vi "Create.vi"(8 "error in (no error)":errorcluster caption="错误输入（无错误）") -> (0 "error out":errorcluster caption="错误输出", 3 "ImageListClass 输出":refnum<class "ImageListClass.lvclass"> caption="DNL_LabVIEW Object out")   [LabVIEW 2013, in "ImageListClass.lvclass"]
uses:
  ImageListClass.lvclass
  System.Windows.Forms
  ImageListClass.lvclass/ImageListClass.ctl
panel:
  in  "ImageListClass 输入":refnum<class "ImageListClass.lvclass"> caption="DNL_LabVIEW Object in"
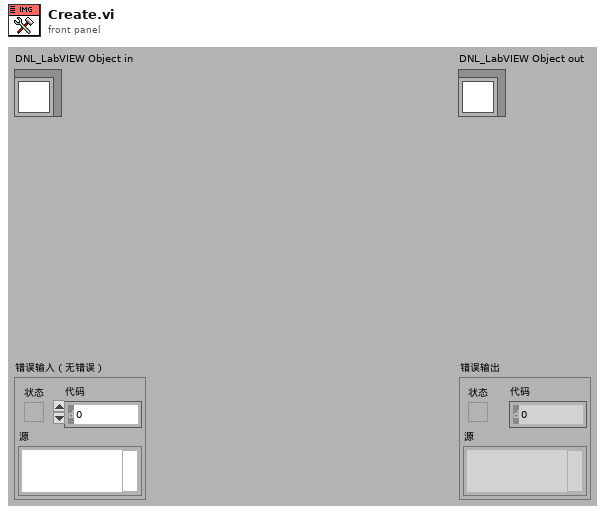
[diagram p1: front panel]
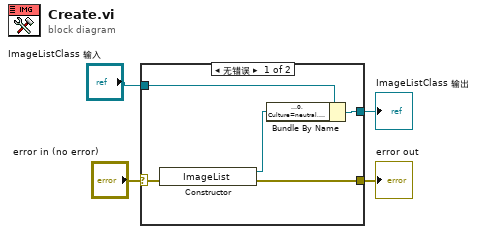
[diagram p0: block diagram]
diagram:
  n1 = case shown="无错误" "error in (no error)" {
    selector: "error in (no error)" -> [w6 w11]
    tunnel: [w5 w11] -> w3
    tunnel: [w8 w10] -> w1
    tunnel: "ImageListClass 输入" -> [w9 w10]
    frame No Error {
      n2 = constructor class="ImageList"(error in=w6) -> (reference out=w7:refnum<k24>, error out=w5:errorcluster)  [unwired: 2 in, 1 out]
      n3 = Bundle By Name(cluster=w9, "ImageList"=w7) -> (w8:refnum<class "ImageListClass.lvclass">)
    }
    frame Error {
    }
  }
  "error out" <- w3
  "ImageListClass 输出" <- w1
